vi "System Monitoring.vi"(7 "Error":errorcluster, 9 "Current FPGA VI Reference":T1, 10 "Refnum in":refnum<k21>) -> (0 "Error":errorcluster, 1 "FPGA Error":errorcluster, 2 "Different Channel Count":bool, 3 "Refnum out":refnum<k21>, 4 "DMA FIFO Full":bool, 6 "Sample Gated":bool)   [LabVIEW 2014]
uses:
  controls/FPGA VI Reference.ctl
  <vilib>/Utility/error.llb/Error Cluster From Error Code.vi
  <vilib>/rvi/errors/niLvFpgaAdjustHostInterfaceError.vi
  <vilib>/rvi/interface/nirviReadWriteControl/nirviReadWriteControl.xnode
  <vilib>/NI_Real-Time Target Support.lvlib
  <resource>/objmgr/nisysapi.rc
  NiFpgaLv.dll
  <vilib>/rvi/interface/Simulation/niFpgaSimulationCallBeginRW.vi
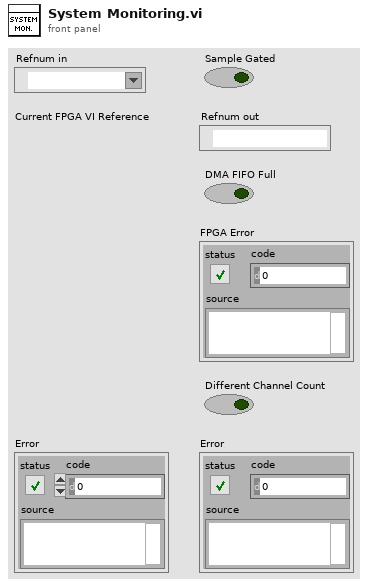
[diagram p1: front panel]
types:
  T1 = typedef "FPGA VI Reference.ctl" = refnum<k20>
  T2 = typedef "NI_Real-Time Target Support.lvlib/RT CPU Load.ctl" = cluster{"Total (%)":dbl, "Time Critical (%)":dbl, "Timed Structures (%)":dbl, "High (%)":dbl, "Above Normal (%)":dbl, "Normal (%)":dbl, "Background (%)":dbl, "Idle (%)":dbl, "ISR (%)":dbl}
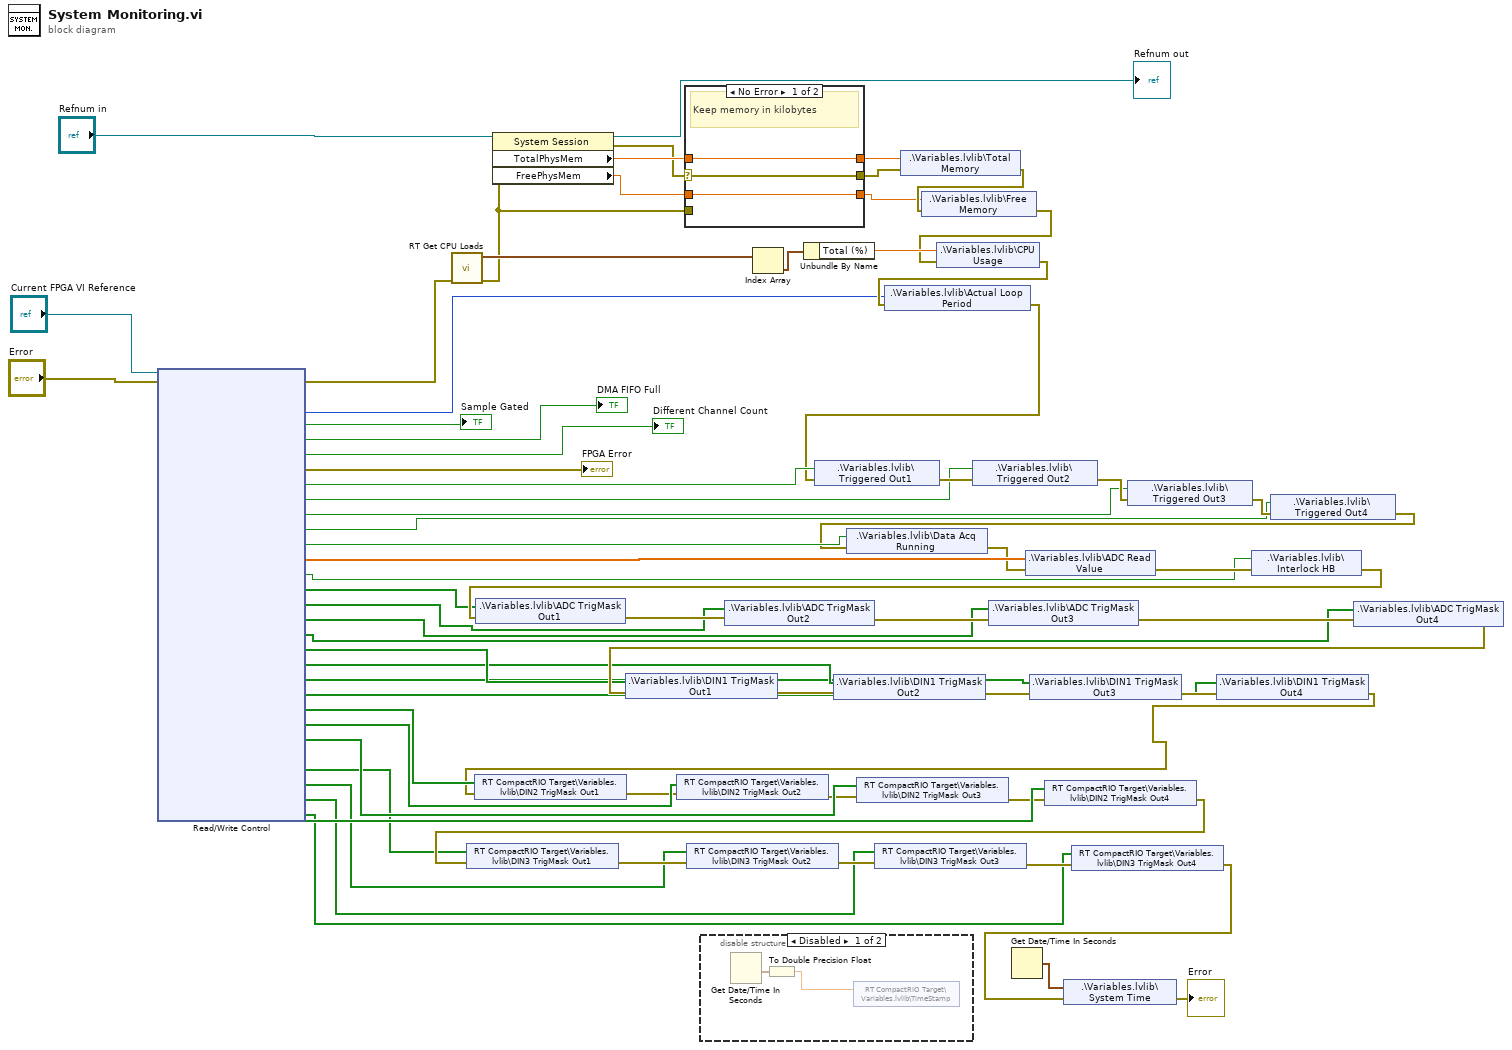
[diagram p0: block diagram]
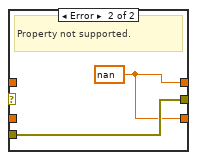
[diagram p3: hidden frame]
diagram:
  n1 = xnode "Read/Write Control"("FPGA VI Reference In"="Current FPGA VI Reference", "error in"="Error") -> ("error out"=w56:errorcluster, "Sample Period (uSec)"=w57:u32, "Sample Gated"=→"Sample Gated":bool, "DMA FIFO Full"=→"DMA FIFO Full":bool, "Different Channel Count"=→"Different Channel Count":bool, "FPGA Error"=→"FPGA Error":errorcluster, "Interlock Out1"=w35:bool, "Interlock Out2"=w34:bool, "Interlock Out3"=w33:bool, "Interlock Out4"=w32:bool, "Data Acq Running"=w51:bool, "Current sample"=w50:sgl[], "Interlock HB"=w12:bool, "ADC TrigMask Out1"=w11:bool[], "ADC TrigMask Out2"=w10:bool[], "ADC TrigMask Out3"=w9:bool[], "ADC TrigMask Out4"=w8:bool[], "DIN1 TrigMask Out1"=w46:bool[], "DIN1 TrigMask Out2"=w42:bool[], "DIN1 TrigMask Out3"=w41:bool[], "DIN1 TrigMask Out4"=w40:bool[], "DIN2 TrigMask Out1"=w31:bool[], "DIN2 TrigMask Out2"=w30:bool[], "DIN2 TrigMask Out3"=w29:bool[], "DIN2 TrigMask Out4"=w28:bool[], "DIN3 TrigMask Out1"=w20:bool[], "DIN3 TrigMask Out2"=w19:bool[], "DIN3 TrigMask Out3"=w18:bool[], "DIN3 TrigMask Out4"=w17:bool[])  [unwired: 2 out]
  n2 = call <vilib>:"RT Get CPU Loads.vi"("error in (no error)"=w56) -> ("error out"=w52:errorcluster, "CPU loads"=w54:T2[])  [unwired: 9 in]
  n3 = property class="System Session"(reference="Refnum in", error in=w52) -> (reference out=→"Refnum out":refnum<k21>, error out=w53:errorcluster, "TotalPhysMem"=w71:dbl, "FreePhysMem"=w2:dbl)
  n4 = case shown="No Error" w53 {
    selector: w53 -> [w75 _]
    tunnel: w71 -> [w74 _]
    tunnel: [w74 w76] -> w69
    tunnel: [w75 w77] -> w70
    tunnel: w52 -> [_ w77]
    tunnel: w2 -> [w73 _]
    tunnel: [w73 w76] -> w1
    frame No Error {
      # "Keep memory in kilobytes"
    }
    frame Error {
      w76 = nan
      # "Property not supported."
    }
  }
  n5 = disable-structure shown="Disabled" {
    frame Disabled {
      n6 = Get Date/Time In Seconds() -> (seconds since 1Jan1904=w79:timestamp)
      n7 = To Double Precision Float(number=w79) -> (double precision float=w78:dbl)
      n8 = shared-variable "RT CompactRIO Target\\Variables.lvlib\\TimeStamp"(w78) -> ()  [unwired: 1 in, 1 out]
    }
    frame Enabled {
    }
  }
  n9 = Index Array(array=w54) -> (element=w55:T2)  [unwired: 1 in]
  n10 = Unbundle By Name(w55) -> ("Total (%)"=w63:dbl)
  n11 = shared-variable ".\\Variables.lvlib\\Total Memory"(w69, error in=w70) -> (error out=w4:errorcluster)
  n12 = shared-variable ".\\Variables.lvlib\\Free Memory"(w1, error in=w4) -> (error out=w3:errorcluster)
  n13 = shared-variable ".\\Variables.lvlib\\CPU Usage"(w63, error in=w3) -> (error out=w68:errorcluster)
  n14 = shared-variable ".\\Variables.lvlib\\Actual Loop Period"(w57, error in=w68) -> (error out=w7:errorcluster)
  n15 = shared-variable ".\\Variables.lvlib\\Triggered Out1"(w35, error in=w7) -> (error out=w39:errorcluster)
  n16 = shared-variable ".\\Variables.lvlib\\Triggered Out2"(w34, error in=w39) -> (error out=w38:errorcluster)
  n17 = Get Date/Time In Seconds() -> (seconds since 1Jan1904=w65:timestamp)
  n18 = shared-variable ".\\Variables.lvlib\\Triggered Out3"(w33, error in=w38) -> (error out=w37:errorcluster)
  n19 = shared-variable ".\\Variables.lvlib\\Triggered Out4"(w32, error in=w37) -> (error out=w36:errorcluster)
  n20 = shared-variable ".\\Variables.lvlib\\Data Acq Running"(w51, error in=w36) -> (error out=w49:errorcluster)
  n21 = shared-variable ".\\Variables.lvlib\\ADC Read Value"(w50, error in=w49) -> (error out=w48:errorcluster)
  n22 = shared-variable ".\\Variables.lvlib\\Interlock HB"(w12, error in=w48) -> (error out=w16:errorcluster)
  n23 = shared-variable ".\\Variables.lvlib\\ADC TrigMask Out1"(w11, error in=w16) -> (error out=w15:errorcluster)
  n24 = shared-variable ".\\Variables.lvlib\\ADC TrigMask Out2"(w10, error in=w15) -> (error out=w14:errorcluster)
  n25 = shared-variable ".\\Variables.lvlib\\ADC TrigMask Out3"(w9, error in=w14) -> (error out=w13:errorcluster)
  n26 = shared-variable ".\\Variables.lvlib\\ADC TrigMask Out4"(w8, error in=w13) -> (error out=w47:errorcluster)
  n27 = shared-variable ".\\Variables.lvlib\\DIN1 TrigMask Out1"(w46, error in=w47) -> (error out=w45:errorcluster)
  n28 = shared-variable ".\\Variables.lvlib\\DIN1 TrigMask Out2"(w42, error in=w45) -> (error out=w44:errorcluster)
  n29 = shared-variable ".\\Variables.lvlib\\DIN1 TrigMask Out3"(w41, error in=w44) -> (error out=w43:errorcluster)
  n30 = shared-variable ".\\Variables.lvlib\\DIN1 TrigMask Out4"(w40, error in=w43) -> (error out=w5:errorcluster)
  n31 = shared-variable "RT CompactRIO Target\\Variables.lvlib\\DIN2 TrigMask Out1"(w31, error in=w5) -> (error out=w27:errorcluster)
  n32 = shared-variable "RT CompactRIO Target\\Variables.lvlib\\DIN2 TrigMask Out2"(w30, error in=w27) -> (error out=w26:errorcluster)
  n33 = shared-variable "RT CompactRIO Target\\Variables.lvlib\\DIN2 TrigMask Out3"(w29, error in=w26) -> (error out=w25:errorcluster)
  n34 = shared-variable "RT CompactRIO Target\\Variables.lvlib\\DIN2 TrigMask Out4"(w28, error in=w25) -> (error out=w21:errorcluster)
  n35 = shared-variable "RT CompactRIO Target\\Variables.lvlib\\DIN3 TrigMask Out1"(w20, error in=w21) -> (error out=w22:errorcluster)
  n36 = shared-variable "RT CompactRIO Target\\Variables.lvlib\\DIN3 TrigMask Out2"(w19, error in=w22) -> (error out=w23:errorcluster)
  n37 = shared-variable "RT CompactRIO Target\\Variables.lvlib\\DIN3 TrigMask Out3"(w18, error in=w23) -> (error out=w24:errorcluster)
  n38 = shared-variable "RT CompactRIO Target\\Variables.lvlib\\DIN3 TrigMask Out4"(w17, error in=w24) -> (error out=w6:errorcluster)
  n39 = shared-variable ".\\Variables.lvlib\\System Time"(w65, error in=w6) -> (error out=→"Error":errorcluster)
